vi "Parse Time from String.vi"(11 "Time string":string) -> (3 "Timestamp":timestamp)   [LabVIEW 2016, in "Packages.lvlib" / "VIPM.lvlib"]
uses:
  VIPM.lvlib
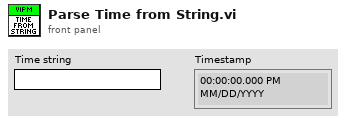
[diagram p1: front panel]
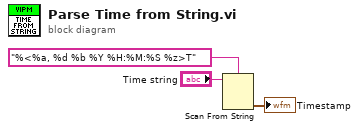
[diagram p0: block diagram]
diagram:
  n1 = Scan From String(format string="%<%a, %d %b %Y %H:%M:%S %z>T", input string="Time string") -> (output 1=→"Timestamp":timestamp)  [unwired: 3 in, 3 out]
